vi "robot_dis.vi"() -> ()   [LabVIEW 2014]
uses:
  <vilib>/robotics/Controls/2D Rangefinder/NI_Robotics_2D Rangefinder.xctl
  <vilib>/Utility/error.llb/DialogType.ctl
  <vilib>/picture/3D Picture Control/Object/Create Object (drawable).vi
  <vilib>/picture/3D Picture Control/Object/Add Object (reference).vi
  <vilib>/picture/3D Picture Control/NI_3D Picture Control.lvlib
panel:
  out "当前拉力":u16
  out "Lidar_two":i32
  in  "选项卡控件":T1
  out "当前速度":u16
  out "当前方向":u8
  in  "开始录像":bool
  in  "上":bool
  in  "下":bool
  in  "左":bool
  in  "加速":bool
  in  "减速":bool
  in  "右":bool
  in  "LED1":u8(slide) step=1 scale=0.0..100.0
  in  "LED2":u8(slide) step=1 scale=0.0..100.0
  in  "LED3":u8(slide) step=1 scale=0.0..100.0
  in  "LED4":u8(slide) step=1 scale=0.0..100.0
  out "控制器":dbl(slide) scale=0.0..100.0
  out "绕线盘":dbl(slide) scale=0.0..100.0 scale format="%.3f"
  out "布尔 3":bool=TRUE
  out "StopChannelRecord":bool
  out "StartChannelRecord":bool
  out "布尔 2":bool
  in  "布尔":bool
  out "StartChannelRealPlay":bool
  in  "Lidar_data":cluster{"数组":dbl[], "数组 2":dbl[][]}
  out "Rangefinder Indicator":cluster{"angle":dbl[], "distance":dbl[][]}(xcontrol)
  out "扫描质量":u8
  out "Lidar_size":u16
  in  "distance":dbl[](array[numeric])
  in  "angle":dbl[](array[numeric])
  out "数值 2":u8 format="%x"
  out "x或y?":u8 format="%x"
  out "x = y?":bool
  out "无符号字节数组 2":u8[](array[numeric])
  out "动力":dbl(slide) scale=0.0..100.0
  out "控制":dbl(slide) scale=0.0..100.0 scale format="%.3f"
  in  "主摄像头":refnum<k7>(container)
  in  "后摄像头":refnum<k7>(container)
  out "Login 2":i32
  out "前摄像头":bool
  out "后摄像头":bool
  out "Login":i32
  in  "前摄像头":refnum<k7>(container)
  in  "AUTO":bool
  in  "上下移动":dbl(slide) scale=-10.0..10.0
  in  "左右移动":dbl(slide) scale=-10.0..10.0
  in  "前后移动":dbl(slide) scale=-10.0..10.0
  in  "缩放":dbl(knob)=2.2771854734286614 scale=0.0..10.0
  out "小车方向":refnum<vi>(3d-picture)
  out "HEANDING":i32
  out "BANK":i32
  out "PITCH":i32
  in  "方向枚举":enum16{"停", "上", "下", "左", "右"}(ring)
  out "和":u8
  out "小车锁定":u8
  out "数据传输":bool
  in  "数据输入":string
  in  "QUIT":bool
  in  "WRITE":bool
  # "TETRAELC--机器人测试平台V0.1"
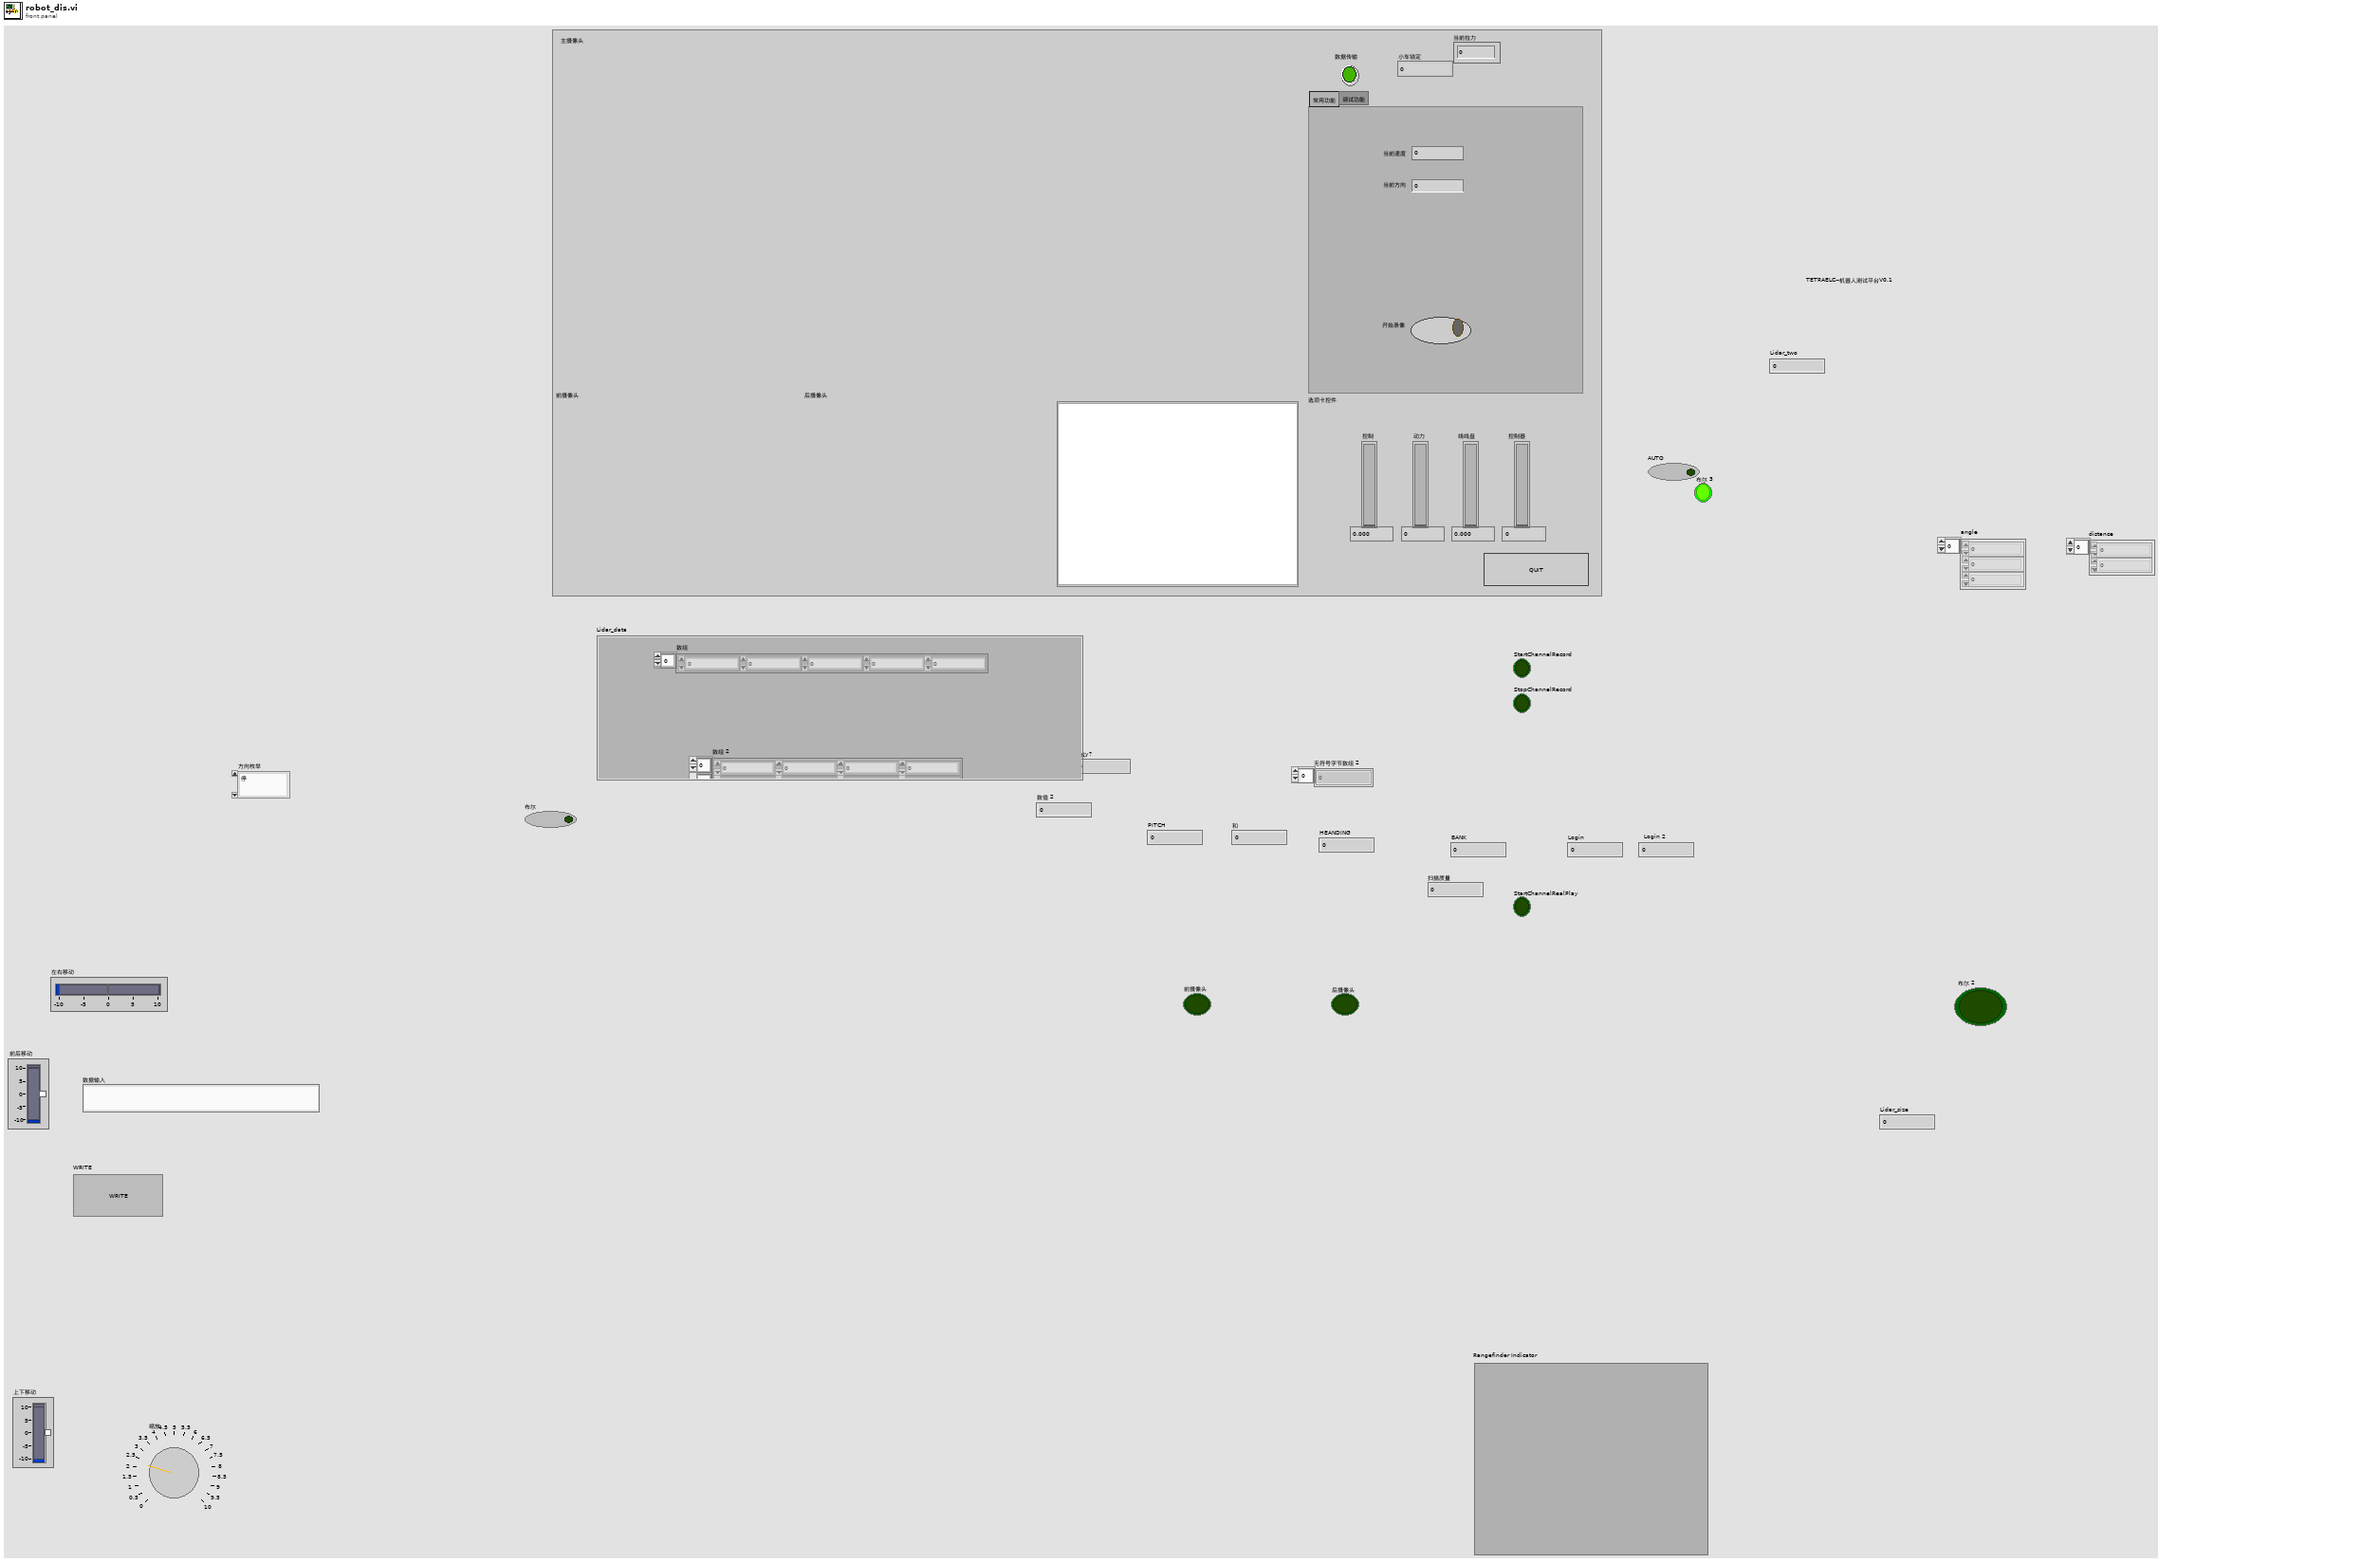
[diagram p1: front panel]
types:
  T1 = typedef "选项卡.ctl" = enum32{"常用功能", "调试功能"}
  T2 = typedef "DialogType.ctl" = u16
  T3 = cluster{"Car_lock":u8, "当前方向":u8, "当前速度\n":u16, "当前拉力":u16}
  T4 = cluster{"PITCH":i32, "BANK":i32, "HEANDING":i32, "X":i32, "Y":i32, "Z":i32}
  T5 = cluster{"quality":u8, "angle":u16, "distance\n":u16}
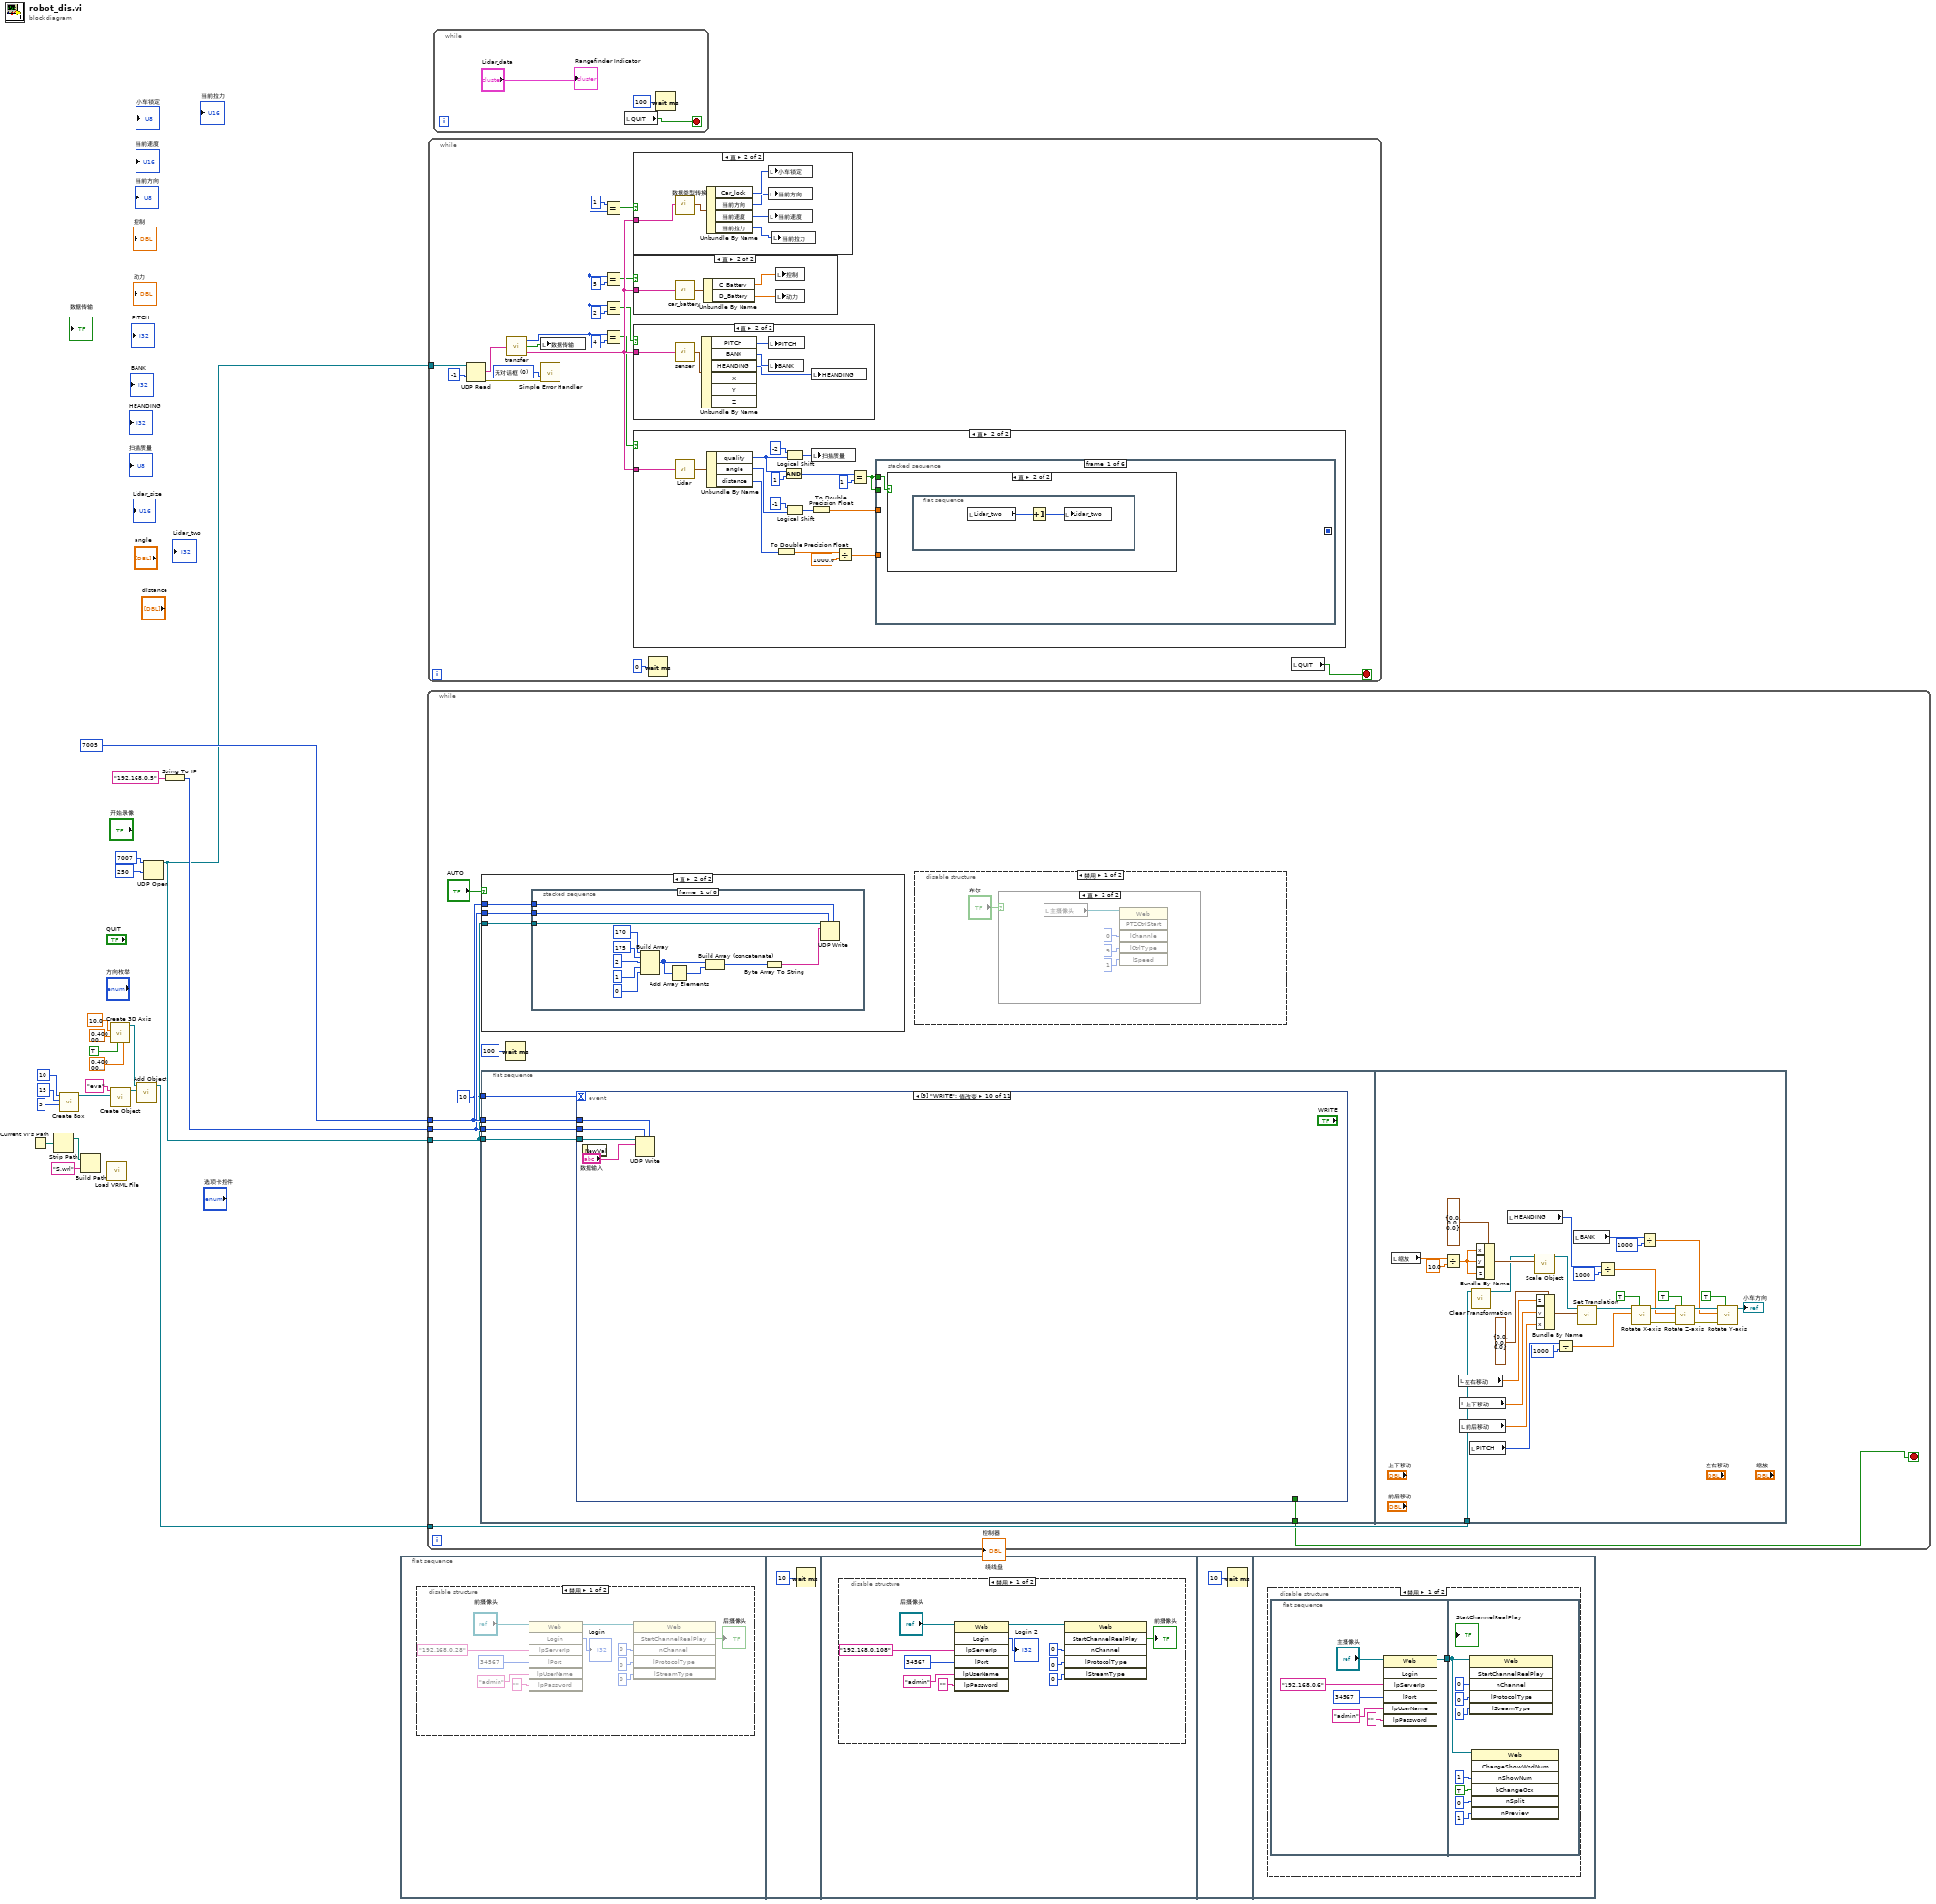
[diagram p0: block diagram]
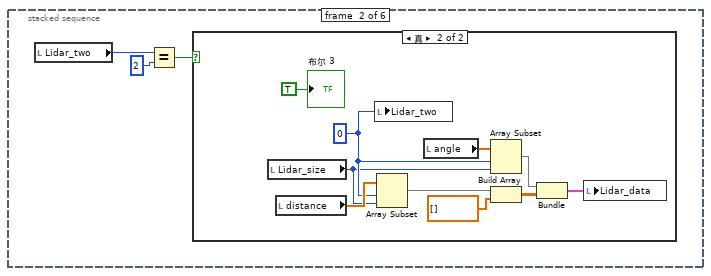
[diagram p4: hidden frame]
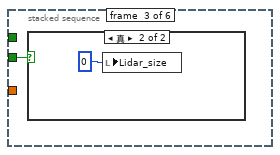
[diagram p6: hidden frame]
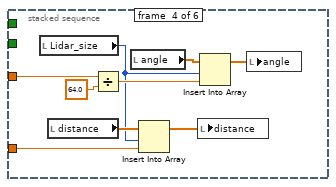
[diagram p8: hidden frame]
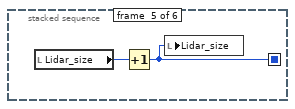
[diagram p9: hidden frame]
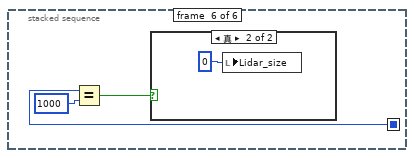
[diagram p10: hidden frame]
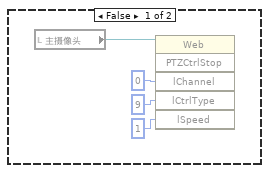
[diagram p18: hidden frame]
diagram:
  n1 = Current VI's Path() -> (path=w6:path)
  n2 = Strip Path(path=w6) -> (stripped path=w5:path)  [unwired: 1 out]
  n3 = call <vilib>:"Create Box.vi"("Length Z"=5, "Length Y"=15, "Length X"=10) -> ("New Box Refnum"=w14:refnum<vi>)  [unwired: 7 in, 1 out]
  n4 = Build Path(base path=w5, name or relative path="S.wrl" ("Name")) -> (appended path=w7:path)
  n5 = call <vilib>:"Load VRML File.vi"("Path"=w7) -> ()  [unwired: 9 in, 2 out]
  n6 = call <vilib>:"Create 3D Axis.vi"("Character Size"=sgl 0.4, "Axis label?"=TRUE, "Radius"=sgl 0.4, "Length"=sgl 10.0) -> ("New Object Refnum"=w9:refnum<vi>)  [unwired: 6 in, 1 out]
  n7 = call-poly <vilib>:"Create Object.vi"("Geometry"=w14, "Name"="eva") -> ("Scene:New Object"=w1:refnum<vi>)  [unwired: 8 in, 1 out]
  n8 = call-poly <vilib>:"Add Object.vi"("New Object In"=w1, "Scene Object In"=w9) -> ("Scene Object Out"=w8:refnum<vi>)  [unwired: 7 in, 2 out]
  n9 = UDP Open(9:250 ("超时毫秒(25000)"), 11:u16 7007 ("本地端口")) -> (port=w2:refnum<k16>)  [unwired: 3 in, 2 out]
  n10 = String To IP(1:"192.168.0.5" ("目标主机")) -> (0:w20:u32)
  n11 = flat-sequence {
    frame #0 {
      n12 = disable-structure shown="禁用" {
        frame Disabled {
          n13 = invoke class="Web" method="Login"(reference="前摄像头", "lpServerIp"="192.168.0.28", "lPort"=34567, "lpUserName"="admin", "lpPassword"="") -> (reference out=w27:refnum<k7>, "Login"=→"Login":i32)  [unwired: 2 in, 5 out]
          n14 = invoke class="Web" method="StartChannelRealPlay"(reference=w27, "nChannel"=0, "lProtocolType"=0, "lStreamType"=0) -> ("StartChannelRealPlay"=→"后摄像头":bool)  [unwired: 2 in, 5 out]
        }
        frame Enabled {
        }
      }
    }
    frame #1 {
      n15 = Wait (ms)(milliseconds to wait=u32 10 ("等待时间（毫秒）")) -> ()  [unwired: 1 out]
    }
    frame #2 {
      n16 = disable-structure shown="禁用" {
        frame Disabled {
          n17 = invoke class="Web" method="Login"(reference="后摄像头", "lpServerIp"="192.168.0.108", "lPort"=34567, "lpUserName"="admin", "lpPassword"="") -> (reference out=w41:refnum<k7>, "Login"=→"Login 2":i32)  [unwired: 2 in, 5 out]
          n18 = invoke class="Web" method="StartChannelRealPlay"(reference=w41, "nChannel"=0, "lProtocolType"=0, "lStreamType"=0) -> ("StartChannelRealPlay"=→"前摄像头":bool)  [unwired: 2 in, 5 out]
        }
        frame Enabled {
        }
      }
    }
    frame #3 {
      n19 = Wait (ms)(milliseconds to wait=u32 10 ("等待时间（毫秒）")) -> ()  [unwired: 1 out]
    }
    frame #4 {
      n20 = disable-structure shown="禁用" {
        frame Disabled {
          n21 = flat-sequence {
            tunnel: [w49] -> w47
            tunnel: w47 -> [w54]
            frame #0 {
              n22 = invoke class="Web" method="Login"(reference="主摄像头", "lpServerIp"="192.168.0.6", "lPort"=34567, "lpUserName"="admin", "lpPassword"="") -> (reference out=w49:refnum<k7>)  [unwired: 2 in, 6 out]
            }
            frame #1 {
              n23 = invoke class="Web" method="StartChannelRealPlay"(reference=w54, "nChannel"=0, "lProtocolType"=0, "lStreamType"=0) -> ()  [unwired: 2 in, 6 out]
              n24 = invoke class="Web" method="ChangeShowWndNum"(reference=w54, "nShowNum"=1, "bChangeOcx"=TRUE, "nSplit"=0, "nPreview"=1) -> ()  [unwired: 2 in, 7 out]
            }
          }
        }
        frame Enabled {
        }
      }
    }
  }
  n25 = while {
    tunnel: w2 -> [w66]
    tunnel: w20 -> [w67]
    tunnel: u16 7005 ("目标端口") -> [w68]
    tunnel: w8 -> [w69]
    stop <- w62 stop-if-true
    n26 = flat-sequence {
      tunnel: 10 -> [w138]
      tunnel: w66 -> [w137]
      tunnel: w67 -> [w136]
      tunnel: w68 -> [w135]
      tunnel: [w134] -> w62
      tunnel: w69 -> [w329]
      frame #0 {
        n27 = event shown="[9] \"WRITE\": 值改变" {
          selector: _ -> [_ _ _ _ _ _ _ _ _ _ _]
          dyn-events: _ -> [_ _ _ _ _ _ _ _ _ _ _]
          timeout: w138 -> [_ _ _ _ _ _ _ _ _ _ _]
          tunnel: w137 -> [_ _ _ w197 w214 w234 w247 w269 w291 w316 w318]
          tunnel: w136 -> [_ _ _ w198 w215 w235 w248 w270 w292 w315 _]
          tunnel: w135 -> [_ _ _ w199 w216 w236 w249 w271 w293 w314 _]
          tunnel: [_ _ _ _ _ _ _ _ _ _ w317] -> w134
          event Timeout {
            n28 = event-data() -> ()  [unwired: 1 in, 1 out]
            n29 = disable-structure shown="禁用" {
              disable-tunnel: _ -> [w155 _]
              frame Disabled {
                n30 = String Subset(string=w155, offset (0)=0 ("长度（剩余）"), length (rest)=100 ("长度（剩余）")) -> (substring=w165:string)
                n31 = String To Byte Array(string=w165) -> (unsigned byte array=w152:u8[])
                "无符号字节数组 2" <- w152
                n32 = Index Array(array=w152, index #1=0 ("索引"), index #2=1 ("索引")) -> (element #1=w143:u8, element #2=w142:u8)
                n33 = for {
                  N: 83 -> [_]
                  tunnel: w152 -> [w172]
                  shift-right: [w167] -> w141
                  shift-left: _ -> [w166]
                  i -> [w171]
                  n34 = Add(x=2, y=w171) -> (x+y=w169:i32)
                  n35 = Index Array(array=w172, index=w169) -> (element=w168:u8)
                  n36 = Exclusive Or(1:w166, 2:w168) -> (0:w167:u8)
                }
                "数值 2" <- w141
                n37 = And(x=w142, y=u8 15) -> (x .and. y?=w145:u8)
                n38 = Logical Shift(y=i16 -4, x=w143) -> (x << y=w158:u8)
                n39 = Logical Shift(y=i16 -4, x=w142) -> (x << y=w156:u8)
                n40 = Equal?(x=w156, y=u8 5) -> (x = y?=w153:bool)
                n41 = Logical Shift(y=i16 4, x=w145) -> (x << y=w147:u8)
                n42 = And(x=w143, y=u8 15) -> (x .and. y?=w146:u8)
                n43 = Equal?(x=w158, y=u8 10) -> (x = y?=w154:bool)
                n44 = And(x=w154, y=w153) -> (x .and. y?=w139:bool)
                n45 = Or(x=w147, y=w146) -> (x .or. y?=w140:u8)
                "x或y?" <- w140
                n46 = case shown="真" w139 {
                  frame False {
                  }
                  frame True {
                    n47 = while {
                      stop <- FALSE stop-if-true
                    }
                    n48 = local read item#-1() -> (w174)
                    n49 = Increment(x=w174) -> (x+1=w173:dbl)
                    n50 = local write item#-1(w173) -> ()
                  }
                }
                n51 = Equal?(x=w140, y=w141) -> ()  [unwired: 1 out]
              }
              frame Enabled {
              }
            }
          }
          event "Lidar_two": Value Change {
            n52 = event-data() -> ()  [unwired: 1 in, 6 out]
            n53 = disable-structure shown="禁用" {
              frame Disabled {
                n54 = local read "Lidar_two"() -> (w178:i32)
                n55 = Equal?(x=w178, y=2) -> (x = y?=w176:bool)
                n56 = case shown="真" w176 {
                  frame False {
                  }
                  frame True {
                  }
                }
              }
              frame Enabled {
              }
            }
          }
          event "开始录像": Value Change {
            n57 = event-data() -> ()  [unwired: 1 in, 6 out]
            n58 = local read "开始录像"() -> (w180:bool)
            n59 = local read "主摄像头"() -> (w181:refnum<k7>)
            n60 = case shown="假" w180 {
              tunnel: w181 -> [w185 w190]
              tunnel: [FALSE ("布尔 2") TRUE ("布尔 2")] -> w179
              frame False {
                n61 = invoke class="Web" method="StopChannelRecord"(reference=w185, "nChannel"=0) -> ("StopChannelRecord"=→"StopChannelRecord":bool)  [unwired: 2 in, 3 out]
              }
              frame True {
                n62 = invoke class="Web" method="StartChannelRecord"(reference=w190, "nChannel"=0, "lpSaveFile"="D:\\record", "nType"=0) -> ("StartChannelRecord"=→"StartChannelRecord":bool)  [unwired: 2 in, 5 out]
              }
            }
            "布尔 2" <- w179
          }
          event "LED1", "LED2", "LED3", "LED4": Value Change {
            n63 = event-data() -> ()  [unwired: 1 in, 6 out]
            n64 = Build Array(u8 170 ("元素"), u8 175 ("元素"), u8 4 ("元素"), u8 8 ("元素"), "LED1", "LED2", "LED3", "LED4") -> (w203:u8[])
            n65 = Add Array Elements(numeric array=w203) -> (sum=w202:u8)
            "和" <- w202
            n66 = Build Array (concatenate)(w203, w202) -> (w201:u8[])
            n67 = Byte Array To String(unsigned byte array=w201) -> (string=w196:string)
            n68 = UDP Write(address=w198, port or service name=w199, connection ID=w197, data in=w196, 9:250 ("超时毫秒(25000)")) -> ()  [unwired: 1 in, 2 out]
          }
          event "加速": Value Change; "减速": Mouse Up {
            n69 = event-data() -> ()  [unwired: 1 in, 4 out]
            n70 = Select(t=i16 1000 ("x"), s="加速", f=i16 -1000) -> (s? t:f=w209:i16)
            n71 = Split Number(x=w209) -> (hi(x)=w213:u8, lo(x)=w212:u8)
            n72 = Build Array(u8 170 ("元素"), u8 175 ("元素"), u8 3 ("元素"), u8 2 ("元素"), w213, w212) -> (w219:u8[])
            n73 = Add Array Elements(numeric array=w219) -> (sum=w218:u8)
            n74 = Build Array (concatenate)(w219, w218) -> (w217:u8[])
            n75 = Byte Array To String(unsigned byte array=w217) -> (string=w224:string)
            n76 = UDP Write(address=w215, port or service name=w216, connection ID=w214, data in=w224) -> ()  [unwired: 2 in, 2 out]
          }
          event "上": Value Change {
            n77 = event-data() -> ()  [unwired: 1 in, 6 out]
            n78 = flat-sequence {
              tunnel: [w241] -> w225
              frame #0 {
                n79 = case shown="真" "上" {
                  frame False {
                    n80 = local write "方向枚举"(enum16{"停", "上", "下", "左", "右"}."停") -> ()
                  }
                  frame True {
                    n81 = local write "方向枚举"(enum16{"停", "上", "下", "左", "右"}."上") -> ()
                  }
                }
              }
              frame #1 {
                n82 = local read "方向枚举"() -> (w240:enum16{"停", "上", "下", "左", "右"})
                n83 = case shown="\"上\", 默认" w240 {
                  tunnel: [u8 0 ("元素") u8 1 ("元素") u8 2 ("元素") u8 3 ("元素") u8 8 ("元素")] -> w241
                  frame "上", Default {
                  }
                  frame "下" {
                  }
                  frame "左" {
                  }
                  frame "右" {
                  }
                  frame "停" {
                  }
                }
              }
            }
            n84 = Build Array(u8 170 ("元素"), u8 175 ("元素"), u8 2 ("元素"), u8 1 ("元素"), w225) -> (w228:u8[])
            n85 = Add Array Elements(numeric array=w228) -> (sum=w227:u8)
            n86 = Build Array (concatenate)(w228, w227) -> (w226:u8[])
            n87 = Byte Array To String(unsigned byte array=w226) -> (string=w233:string)
            n88 = UDP Write(address=w235, port or service name=w236, connection ID=w234, data in=w233) -> ()  [unwired: 2 in, 2 out]
          }
          event "下": Value Change {
            n89 = event-data() -> ()  [unwired: 1 in, 6 out]
            n90 = flat-sequence {
              tunnel: [w263] -> w250
              frame #0 {
                n91 = case shown="真" "下" {
                  frame False {
                    n92 = local write "方向枚举"(enum16{"停", "上", "下", "左", "右"}."停") -> ()
                  }
                  frame True {
                    n93 = local write "方向枚举"(enum16{"停", "上", "下", "左", "右"}."下") -> ()
                  }
                }
              }
              frame #1 {
                n94 = local read "方向枚举"() -> (w262:enum16{"停", "上", "下", "左", "右"})
                n95 = case shown="\"上\", 默认" w262 {
                  tunnel: [u8 0 ("元素") u8 1 ("元素") u8 2 ("元素") u8 3 ("元素") u8 8 ("元素")] -> w263
                  frame "上", Default {
                  }
                  frame "下" {
                  }
                  frame "左" {
                  }
                  frame "右" {
                  }
                  frame "停" {
                  }
                }
              }
            }
            n96 = Build Array(u8 170 ("元素"), u8 175 ("元素"), u8 2 ("元素"), u8 1 ("元素"), w250) -> (w253:u8[])
            n97 = Add Array Elements(numeric array=w253) -> (sum=w252:u8)
            n98 = Build Array (concatenate)(w253, w252) -> (w251:u8[])
            n99 = Byte Array To String(unsigned byte array=w251) -> (string=w258:string)
            n100 = UDP Write(address=w248, port or service name=w249, connection ID=w247, data in=w258) -> ()  [unwired: 2 in, 2 out]
          }
          event "左": Value Change {
            n101 = event-data() -> ()  [unwired: 1 in, 6 out]
            n102 = flat-sequence {
              tunnel: [w285] -> w272
              frame #0 {
                n103 = case shown="真" "左" {
                  frame False {
                    n104 = local write "方向枚举"(enum16{"停", "上", "下", "左", "右"}."停") -> ()
                  }
                  frame True {
                    n105 = local write "方向枚举"(enum16{"停", "上", "下", "左", "右"}."左") -> ()
                  }
                }
              }
              frame #1 {
                n106 = local read "方向枚举"() -> (w284:enum16{"停", "上", "下", "左", "右"})
                n107 = case shown="\"上\", 默认" w284 {
                  tunnel: [u8 0 ("元素") u8 1 ("元素") u8 2 ("元素") u8 3 ("元素") u8 8 ("元素")] -> w285
                  frame "上", Default {
                  }
                  frame "下" {
                  }
                  frame "左" {
                  }
                  frame "右" {
                  }
                  frame "停" {
                  }
                }
              }
            }
            n108 = Build Array(u8 170 ("元素"), u8 175 ("元素"), u8 2 ("元素"), u8 1 ("元素"), w272) -> (w275:u8[])
            n109 = Add Array Elements(numeric array=w275) -> (sum=w274:u8)
            n110 = Build Array (concatenate)(w275, w274) -> (w273:u8[])
            n111 = Byte Array To String(unsigned byte array=w273) -> (string=w280:string)
            n112 = UDP Write(address=w270, port or service name=w271, connection ID=w269, data in=w280) -> ()  [unwired: 2 in, 2 out]
          }
          event "右": Value Change {
            n113 = event-data() -> ()  [unwired: 1 in, 6 out]
            n114 = flat-sequence {
              tunnel: [w307] -> w294
              frame #0 {
                n115 = case shown="真" "右" {
                  frame False {
                    n116 = local write "方向枚举"(enum16{"停", "上", "下", "左", "右"}."停") -> ()
                  }
                  frame True {
                    n117 = local write "方向枚举"(enum16{"停", "上", "下", "左", "右"}."右") -> ()
                  }
                }
              }
              frame #1 {
                n118 = local read "方向枚举"() -> (w306:enum16{"停", "上", "下", "左", "右"})
                n119 = case shown="\"上\", 默认" w306 {
                  tunnel: [u8 0 ("元素") u8 1 ("元素") u8 2 ("元素") u8 3 ("元素") u8 8 ("元素")] -> w307
                  frame "上", Default {
                  }
                  frame "下" {
                  }
                  frame "左" {
                  }
                  frame "右" {
                  }
                  frame "停" {
                  }
                }
              }
            }
            n120 = Build Array(u8 170 ("元素"), u8 175 ("元素"), u8 2 ("元素"), u8 1 ("元素"), w294) -> (w297:u8[])
            n121 = Add Array Elements(numeric array=w297) -> (sum=w296:u8)
            n122 = Build Array (concatenate)(w297, w296) -> (w295:u8[])
            n123 = Byte Array To String(unsigned byte array=w295) -> (string=w302:string)
            n124 = UDP Write(address=w292, port or service name=w293, connection ID=w291, data in=w302) -> ()  [unwired: 2 in, 2 out]
          }
          event "WRITE": Value Change {
            n125 = event-data() -> ()  [unwired: 1 in, 1 out]
            n126 = UDP Write(address=w315, port or service name=w314, connection ID=w316, data in="数据输入") -> ()  [unwired: 2 in, 2 out]
          }
          event "QUIT": Value Change {
            n127 = event-data() -> ()  [unwired: 1 in, 1 out]
            n128 = flat-sequence {
              tunnel: w318 -> [w322]
              tunnel: [TRUE] -> w317
              frame #0 {
                n129 = local read "主摄像头"() -> (w319:refnum<k7>)
                n130 = UDP Close(connection ID=w322) -> ()  [unwired: 1 in, 2 out]
                n131 = local read "后摄像头"() -> (w320:refnum<k7>)
                n132 = local read "前摄像头"() -> (w321:refnum<k7>)
                n133 = invoke class="Web" method="StopRealPlayAll"(reference=w319) -> ()  [unwired: 2 in, 3 out]
                n134 = invoke class="Web" method="StopRealPlayAll"(reference=w320) -> ()  [unwired: 2 in, 3 out]
                n135 = invoke class="Web" method="StopRealPlayAll"(reference=w321) -> ()  [unwired: 2 in, 3 out]
              }
              frame #1 {
              }
            }
          }
        }
      }
      frame #1 {
        n136 = local read "缩放"() -> (w348:dbl)
        n137 = Divide(x=w348, y=10.0) -> (x/y=w352:dbl)
        n138 = local read "左右移动"() -> (w347:dbl)
        n139 = local read "上下移动"() -> (w346:dbl)
        n140 = local read "前后移动"() -> (w345:dbl)
        n141 = local read "PITCH"() -> (w326:i32)
        n142 = call <vilib>:"Clear Transformation.vi"("Object Refnum In"=w329) -> ("Object Refnum Out"=w324:refnum<vi>)  [unwired: 9 in, 1 out]
        n143 = Bundle By Name(cluster=cluster{"x":dbl, "y":dbl, "z":dbl} {"x"=0.0, "y"=0.0, "z"=0.0}, "x"=w352, "y"=w352, "z"=w352) -> (w325:cluster{"x":dbl, "y":dbl, "z":dbl})
        n144 = local read "HEANDING"() -> (w327:i32)
        n145 = call <vilib>:"Scale Object.vi"("Scale"=w325, "Scene.Object In"=w324) -> ("Scene.Object Out"=w354:refnum<vi>)  [unwired: 8 in, 1 out]
        n146 = Bundle By Name(cluster=cluster{"x":dbl, "y":dbl, "z":dbl} {"x"=0.0, "y"=0.0, "z"=0.0}, "z"=w347, "y"=w346, "x"=w345) -> (w351:cluster{"x":dbl, "y":dbl, "z":dbl})
        n147 = Divide(x=w326, y=1000) -> (x/y=w332:dbl)
        n148 = local read "BANK"() -> (w328:i32)
        n149 = call <vilib>:"Set Translation.vi"("Translation"=w351, "Scene Object"=w354) -> ("Translated Object"=w342:refnum<vi>)  [unwired: 8 in, 1 out]
        n150 = Divide(x=w327, y=1000) -> (x/y=w333:dbl)
        n151 = call <vilib>:"Rotate X-axis.vi"("Relative?"=TRUE, "angle"=w332, "Scene Object In"=w342) -> ("error out"=w341:errorcluster, "Scene Object Out"=w340:refnum<vi>)  [unwired: 7 in]
        n152 = Divide(x=w328, y=1000) -> (x/y=w331:dbl)
        n153 = call <vilib>:"Rotate Z-axis.vi"("Relative?"=TRUE, "error in (no error)"=w341, "angle"=w333, "Scene Object In"=w340) -> ("error out"=w337:errorcluster, "Scene Object Out"=w336:refnum<vi>)  [unwired: 6 in]
        n154 = call <vilib>:"Rotate Y-axis.vi"("Relative?"=TRUE, "error in (no error)"=w337, "angle"=w331, "Scene Object In"=w336) -> ("Scene Object Out"=→"小车方向":refnum<vi>)  [unwired: 6 in, 1 out]
      }
    }
    n155 = case shown="真" "AUTO" {
      tunnel: w68 -> [_ w81]
      tunnel: w67 -> [_ w80]
      tunnel: w66 -> [_ w79]
      frame False {
      }
      frame True {
        n156 = stacked-sequence {
          tunnel: w81 -> [w84 _ w95 _ w109 _ w122 _]
          tunnel: w80 -> [w83 _ w96 _ w110 _ w123 _]
          tunnel: w79 -> [w82 _ w97 _ w111 _ w121 _]
          frame #0 {
            n157 = Build Array(u8 170 ("元素"), u8 175 ("元素"), u8 2 ("元素"), u8 1 ("元素"), u8 0 ("元素")) -> (w88:u8[])
            n158 = Add Array Elements(numeric array=w88) -> (sum=w87:u8)
            n159 = Build Array (concatenate)(w88, w87) -> (w86:u8[])
            n160 = Byte Array To String(unsigned byte array=w86) -> (string=w93:string)
            n161 = UDP Write(address=w83, port or service name=w84, connection ID=w82, data in=w93) -> ()  [unwired: 2 in, 2 out]
          }
          frame #1 {
            n162 = Wait (ms)(milliseconds to wait=u32 3000 ("等待时间（毫秒）")) -> ()  [unwired: 1 out]
          }
          frame #2 {
            n163 = Build Array(u8 170 ("元素"), u8 175 ("元素"), u8 2 ("元素"), u8 1 ("元素"), u8 8 ("元素")) -> (w101:u8[])
            n164 = Add Array Elements(numeric array=w101) -> (sum=w100:u8)
            n165 = Build Array (concatenate)(w101, w100) -> (w99:u8[])
            n166 = Byte Array To String(unsigned byte array=w99) -> (string=w106:string)
            n167 = UDP Write(address=w96, port or service name=w95, connection ID=w97, data in=w106) -> ()  [unwired: 2 in, 2 out]
          }
          frame #3 {
            n168 = Wait (ms)(milliseconds to wait=u32 1000 ("等待时间（毫秒）")) -> ()  [unwired: 1 out]
          }
          frame #4 {
            n169 = Build Array(u8 170 ("元素"), u8 175 ("元素"), u8 2 ("元素"), u8 1 ("元素"), u8 1 ("元素")) -> (w115:u8[])
            n170 = Add Array Elements(numeric array=w115) -> (sum=w114:u8)
            n171 = Build Array (concatenate)(w115, w114) -> (w113:u8[])
            n172 = Byte Array To String(unsigned byte array=w113) -> (string=w119:string)
            n173 = UDP Write(address=w110, port or service name=w109, connection ID=w111, data in=w119) -> ()  [unwired: 2 in, 2 out]
          }
          frame #5 {
            n174 = Wait (ms)(milliseconds to wait=u32 3000 ("等待时间（毫秒）")) -> ()  [unwired: 1 out]
          }
          frame #6 {
            n175 = Build Array(u8 170 ("元素"), u8 175 ("元素"), u8 2 ("元素"), u8 1 ("元素"), u8 8 ("元素")) -> (w127:u8[])
            n176 = Add Array Elements(numeric array=w127) -> (sum=w126:u8)
            n177 = Build Array (concatenate)(w127, w126) -> (w125:u8[])
            n178 = Byte Array To String(unsigned byte array=w125) -> (string=w132:string)
            n179 = UDP Write(address=w123, port or service name=w122, connection ID=w121, data in=w132) -> ()  [unwired: 2 in, 2 out]
          }
          frame #7 {
            n180 = Wait (ms)(milliseconds to wait=u32 1000 ("等待时间（毫秒）")) -> ()  [unwired: 1 out]
          }
        }
      }
    }
    n181 = Wait (ms)(milliseconds to wait=u32 100 ("等待时间（毫秒）")) -> ()  [unwired: 1 out]
    n182 = disable-structure shown="禁用" {
      frame Disabled {
        n183 = case shown="真" "布尔" {
          frame False {
            n184 = local read "主摄像头"() -> (w74:refnum<k7>)
            n185 = invoke class="Web" method="PTZCtrlStop"(reference=w74, "lChannel"=0, "lCtrlType"=9, "lSpeed"=1) -> ()  [unwired: 2 in, 6 out]
          }
          frame True {
            n186 = local read "主摄像头"() -> (w78:refnum<k7>)
            n187 = invoke class="Web" method="PTZCtrlStart"(reference=w78, "lChannle"=0, "lCtrlType"=9, "lSpeed"=1) -> ()  [unwired: 2 in, 6 out]
          }
        }
      }
      frame Enabled {
      }
    }
  }
  n188 = while {
    tunnel: w2 -> [w358]
    stop <- w355 stop-if-true
    w361 = T2 0 items=["无对话框", "确定信息", "继续或停止信息", "确定信息＋警告", "继续/停止+警告"] ("type of dialog (OK msg:1)")
    n189 = UDP Read(connection ID=w358, timeout ms (25000)=-1 ("超时毫秒(25000)")) -> (data out=w362:string, error out=w360:errorcluster)  [unwired: 2 in, 3 out]
    n190 = call "transfer.vi"("输入"=w362) -> ("数值"=w369:u8, "布尔"=w357:bool, "输出"=w372:string)
    n191 = local write "数据传输"(w357) -> ()
    n192 = call <vilib>:"Simple Error Handler.vi"("type of dialog (OK msg:1)"=w361, "error in (no error)"=w360) -> ()  [unwired: 3 in, 5 out]
    n193 = Equal?(x=u8 1, y=w369) -> (x = y?=w364:bool)
    n194 = Equal?(x=w369, y=u8 5 ("x")) -> (x = y?=w368:bool)
    n195 = Equal?(x=w369, y=u8 2 ("x")) -> (x = y?=w366:bool)
    n196 = Equal?(x=w369, y=u8 4 ("x")) -> (x = y?=w371:bool)
    n197 = case shown="真" w364 {
      tunnel: w372 -> [_ w433]
      frame False {
      }
      frame True {
        n198 = call "数据类型转换.vi"("read buffer"=w433) -> ("输出簇"=w432:T3)
        n199 = Unbundle By Name(w432) -> ("Car_lock"=w431:u8, "当前方向"=w430:u8, "当前速度"=w429:u16, "当前拉力"=w428:u16)
        n200 = local write "小车锁定"(w431) -> ()
        n201 = local write "当前方向"(w430) -> ()
        n202 = local write "当前速度"(w429) -> ()
        n203 = local write "当前拉力"(w428) -> ()
      }
    }
    n204 = case shown="真" w368 {
      tunnel: w372 -> [_ w437]
      frame False {
      }
      frame True {
        n205 = call "car_battery.vi"("read buffer"=w437) -> ("输出簇"=w436:cluster{"C_Battery":dbl, "D_Battery\n":dbl})
        n206 = Unbundle By Name(w436) -> ("C_Battery"=w435:dbl, "D_Battery"=w434:dbl)
        n207 = local write "控制"(w435) -> ()
        n208 = local write "动力"(w434) -> ()
      }
    }
    n209 = case shown="真" w366 {
      tunnel: w372 -> [_ w427]
      frame False {
      }
      frame True {
        n210 = call "senser.vi"("read buffer"=w427) -> ("输出簇"=w426:T4)
        n211 = Unbundle By Name(w426) -> ("PITCH"=w425:i32, "BANK"=w424:i32, "HEANDING"=w423:i32)  [unwired: 3 out]
        n212 = local write "PITCH"(w425) -> ()
        n213 = local write "BANK"(w424) -> ()
        n214 = local write "HEANDING"(w423) -> ()
      }
    }
    n215 = case shown="真" w371 {
      tunnel: w372 -> [_ w389]
      frame False {
      }
      frame True {
        n216 = call "Lidar.vi"("read buffer"=w389) -> ("输出簇"=w388:T5)
        n217 = Unbundle By Name(w388) -> ("quality"=w380:u8, "angle"=w384:u16, "distance"=w376:u16)
        n218 = To Double Precision Float(number=w376) -> (double precision float=w375:dbl)
        n219 = And(x=w380, y=u8 1) -> (x .and. y?=w379:u8)
        n220 = Logical Shift(y=i16 -2, x=w380) -> (x << y=w385:u8)
        n221 = Logical Shift(y=i16 -1, x=w384) -> (x << y=w383:u16)
        n222 = local write "扫描质量"(w385) -> ()
        n223 = To Double Precision Float(number=w383) -> (double precision float=w381:dbl)
        n224 = Divide(x=w375, y=1000.0) -> (x/y=w373:dbl)
        n225 = Equal?(x=w379, y=u8 1) -> (x = y?=w377:bool)
        n226 = stacked-sequence {
          seq-local: [_ _ _ _ w417 _] -> [_ _ _ _ _ w420]
          tunnel: w377 -> [w390 _ _ _ _ _]
          tunnel: w377 -> [_ _ w406 _ _ _]
          tunnel: w381 -> [_ _ _ w413 _ _]
          tunnel: w373 -> [_ _ _ w408 _ _]
          frame #0 {
            n227 = case shown="真" w390 {
              frame False {
              }
              frame True {
                n228 = flat-sequence {
                  frame #0 {
                    n229 = local read "Lidar_two"() -> (w392:i32)
                    n230 = Increment(x=w392) -> (x+1=w391:i32)
                    n231 = local write "Lidar_two"(w391) -> ()
                  }
                }
              }
            }
          }
          frame #1 {
            n232 = local read "Lidar_two"() -> (w395:i32)
            n233 = Equal?(x=w395, y=2) -> (x = y?=w393:bool)
            n234 = case shown="真" w393 {
              frame False {
              }
              frame True {
                w403 = 0 ("Lidar_two")
                n235 = local read "Lidar_size"() -> (w402:u16)
                n236 = local read "distance"() -> (w404:dbl[])
                n237 = local write "Lidar_two"(w403) -> ()
                n238 = Array Subset(array=w404, index=w403, length=w402) -> (w401:dbl[])
                n239 = local read "angle"() -> (w405:dbl[])
                n240 = Array Subset(array=w405, index=w403, length=w402) -> (w399:dbl[])
                n241 = Build Array(w401, dbl[] [] ("元素")) -> (w398:dbl[][])
                n242 = Bundle(w399, w398) -> (w396:cluster{dbl[], dbl[][]})  [unwired: 1 in]
                n243 = local write "Lidar_data"(w396) -> ()
                "布尔 3" <- TRUE
              }
            }
          }
          frame #2 {
            n244 = case shown="真" w406 {
              frame False {
              }
              frame True {
                n245 = local write "Lidar_size"(u8 0 ("Lidar_size")) -> ()
              }
            }
          }
          frame #3 {
            n246 = local read "Lidar_size"() -> (w409:u16)
            n247 = local read "distance"() -> (w410:dbl[])
            n248 = Divide(x=w413, y=64.0) -> (x/y=w412:dbl)
            n249 = local read "angle"() -> (w416:dbl[])
            n250 = Insert Into Array(array=w410, index=w409, new element=w408) -> (w411:dbl[])
            n251 = local write "distance"(w411) -> ()
            n252 = Insert Into Array(array=w416, index=w409, new element=w412) -> (w415:dbl[])
            n253 = local write "angle"(w415) -> ()
          }
          frame #4 {
            n254 = local read "Lidar_size"() -> (w418:u16)
            n255 = Increment(x=w418) -> (x+1=w417:u16)
            n256 = local write "Lidar_size"(w417) -> ()
          }
          frame #5 {
            n257 = Equal?(x=w420, y=u16 1000) -> (x = y?=w419:bool)
            n258 = case shown="真" w419 {
              frame False {
              }
              frame True {
                n259 = local write "Lidar_size"(u16 0 ("Lidar_size")) -> ()
              }
            }
          }
        }
      }
    }
    n260 = Wait (ms)(milliseconds to wait=u32 0 ("等待时间（毫秒）")) -> ()  [unwired: 1 out]
    n261 = local read "QUIT"() -> (w355:bool)
  }
  n262 = while {
    stop <- w438 stop-if-true
    n263 = local read "QUIT"() -> (w438:bool)
    n264 = Wait (ms)(milliseconds to wait=u32 100 ("等待时间（毫秒）")) -> ()  [unwired: 1 out]
    "Rangefinder Indicator" <- "Lidar_data"
  }
